vi "set Light Direction.vi"(10 "Light Direction":T1, 11 "Scene in":refnum<class "Scene.lvclass">) -> (3 "Scene out":refnum<class "Scene.lvclass">)   [LabVIEW 2020, in "Scene.lvclass"]
uses:
  Scene.lvclass
  Scene.lvclass/Scene.ctl
  Graphics/Libraries/3D/Vector 3D.ctl
  Graphics/Libraries/3D/3D.lvlib
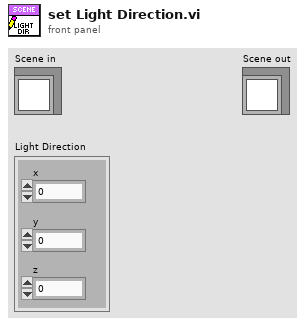
[diagram p1: front panel]
types:
  T1 = typedef "3D.lvlib/Vector 3D.ctl" = cluster{"x":sgl, "y":sgl, "z":sgl}
  T2 = typedef "3D.lvlib/Object.ctl" = cluster{"Triangles":T3[], "Transform":T9, "Name":string, "Alpha Blending Enabled":bool, "Alpha":dbl, "Turntable Enabled":bool, "Material":T6}
  T3 = typedef "3D.lvlib/Triangle.ctl" = cluster{"Vertex 1":T4, "Vertex 2":T4, "Vertex 3":T4, "Alpha":dbl, "Alpha Blending Enabled":bool, "Colour":u32, "Material":T6}
  T4 = typedef "3D.lvlib/Vertex.ctl" = cluster{"Position":T1, "UV":T5, "Colour":u32}
  T5 = typedef "Raster.lvlib/UV.ctl" = cluster{"u":sgl, "v":sgl}
  T6 = typedef "3D.lvlib/Material.ctl" = cluster{"Diffuse Colour":u32, "Texture":T7}
  T7 = typedef "Raster.lvlib/Texture.ctl" = cluster{"Pixels":refnum<data-value>, "Size":T8}
  T8 = typedef "Raster.lvlib/Rectangle Dimensions.ctl" = cluster{"Width":u32, "Height":u32}
  T9 = typedef "3D.lvlib/Transform.ctl" = cluster{"Position":T1, "Rotation":T1, "Scale":T1}
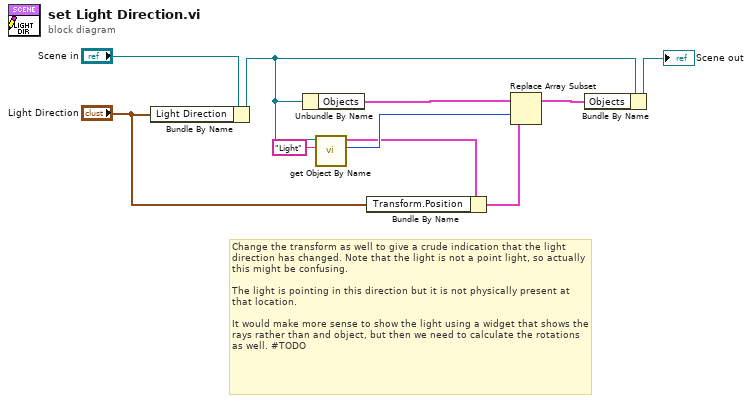
[diagram p0: block diagram]
diagram:
  # "Change the transform as well to give a crude indication that the light direction has changed. Note that the light is not a point light, so actually this might be confusing.\n\nThe light is pointing in this direction but it is not physically present at that location.\n\nIt would make more sense to show the light using a widget that shows the rays rather than and object, but then we need to calculate the rotations as well. #TODO"
  n1 = Bundle By Name(cluster="Scene in", "Light Direction"="Light Direction") -> (w4:refnum<class "Scene.lvclass">)
  n2 = Unbundle By Name(w4) -> ("Objects"=w9:T2[])
  n3 = call "get Object By Name.vi"("Name"="Light", "Scene in"=w4) -> ("Index"=w8:i32, "Object"=w7:T2)  [unwired: 8 in]
  n4 = Bundle By Name(cluster=w7, "Transform.Position"="Light Direction") -> (w5:T2)
  n5 = Replace Array Subset(array=w9, new element=w5, index=w8) -> (w3:T2[])
  n6 = Bundle By Name(cluster=w4, "Objects"=w3) -> (→"Scene out":refnum<class "Scene.lvclass">)
